vi "CAlex2_rtDisplay.vi"(8 "Cloest Pt":dbl[](array[numeric]), 9 "PrevTraj":dbl[][](array[numeric]), 10 "TargetTraj":dbl[][](array[numeric]), 11 "JointLoc":dbl[][](array[numeric])) -> (3 "new picture":picture)   [LabVIEW 2016, in "CAlex2.lvclass"]
uses:
  CAlex2/CAlex2.lvclass
panel:
  in  "Scale (1) and Offset (0,0)":cluster{"x":i16, "y":i16, "Scale":dbl}={"x"=0, "y"=0, "Scale"=1.0}
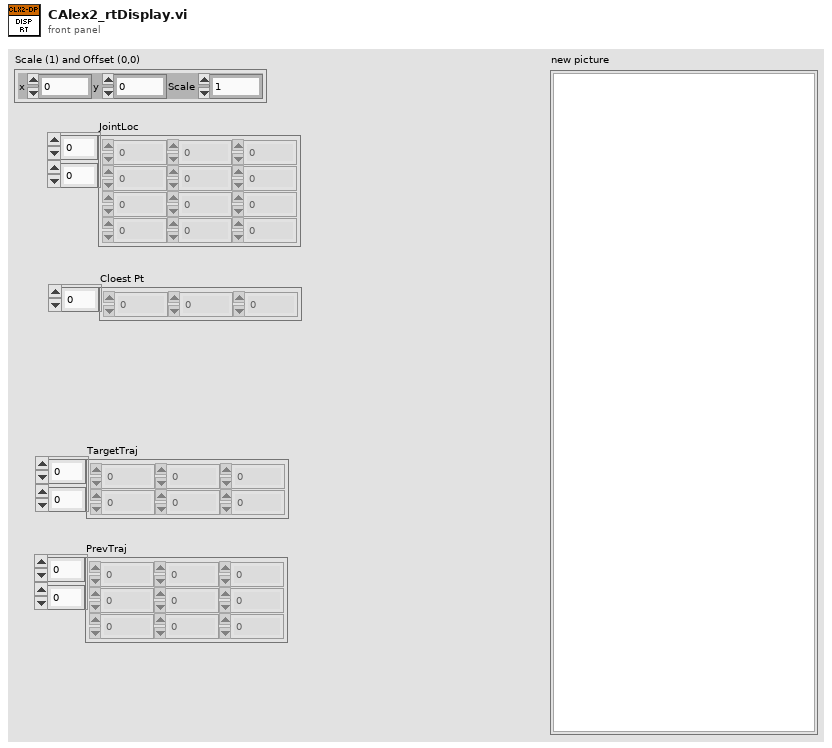
[diagram p1: front panel]
types:
  T1 = cluster{"Width":u16, "Style":enum32{"Solid", "Dash", "Dot", "DashDot", "DashDotDot"}}
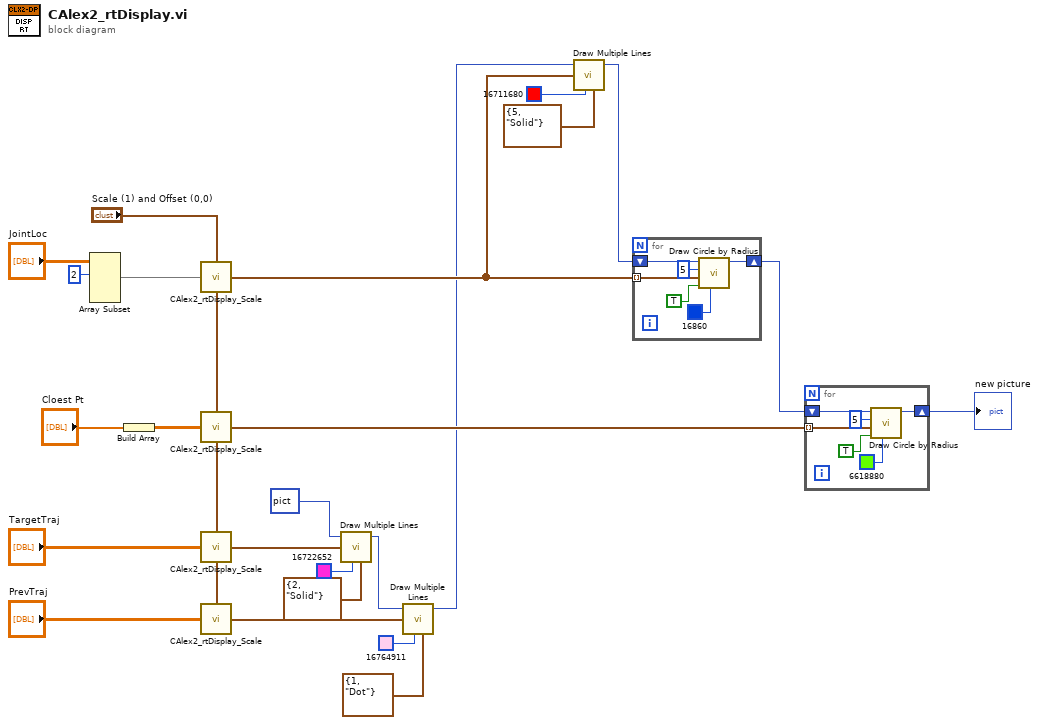
[diagram p0: block diagram]
diagram:
  n1 = Array Subset(array="JointLoc", index (row)=2 ("index")) -> (w9:dbl[][])  [unwired: 3 in]
  n2 = Build Array("Cloest Pt") -> (w6:dbl[][])
  n3 = call "CAlex2_rtDisplay_Scale.vi"("Scale (1) and Offset (0,0)"="Scale (1) and Offset (0,0)", "Input XYZ array"=w9) -> ("Output XY array"=w17:cluster{i16, i16}[])  [unwired: 2 in]
  n4 = call "CAlex2_rtDisplay_Scale.vi"("Scale (1) and Offset (0,0)"="Scale (1) and Offset (0,0)", "Input XYZ array"=w6) -> ("Output XY array"=w5:cluster{i16, i16}[])  [unwired: 2 in]
  n5 = call "CAlex2_rtDisplay_Scale.vi"("Scale (1) and Offset (0,0)"="Scale (1) and Offset (0,0)", "Input XYZ array"="TargetTraj") -> ("Output XY array"=w22:cluster{i16, i16}[])  [unwired: 2 in]
  n6 = call "CAlex2_rtDisplay_Scale.vi"("Scale (1) and Offset (0,0)"="Scale (1) and Offset (0,0)", "Input XYZ array"="PrevTraj") -> ("Output XY array"=w21:cluster{i16, i16}[])  [unwired: 2 in]
  n7 = call <vilib>:"Draw Multiple Lines.vi"("picture"=picture data[5B] ("blank picture"), "line endpoints"=w22, "color(black)"=u32 16722652, "pen"=T1 {"Width"=2, "Style"=enum."Solid"}) -> ("new picture"=w20:picture)  [unwired: 5 in]
  n8 = call <vilib>:"Draw Multiple Lines.vi"("picture"=w20, "line endpoints"=w21, "color(black)"=u32 16764911, "pen"=T1 {"Width"=1, "Style"=enum."Dot"}) -> ("new picture"=w2:picture)  [unwired: 5 in]
  n9 = call <vilib>:"Draw Multiple Lines.vi"("picture"=w2, "line endpoints"=w17, "color(black)"=u32 16711680, "pen"=T1 {"Width"=5, "Style"=enum."Solid"}) -> ("new picture"=w16:picture)  [unwired: 5 in]
  n10 = for {
    tunnel: w17 -> [w30] mode=indexing
    shift-right: [w28] -> w4
    shift-left: w16 -> [w29]
    n11 = call <vilib>:"Draw Circle by Radius.vi"("color(black)"=u32 16860, "fill?(F)"=TRUE, "pixel center"=w30, "radius"=i16 5, "picture"=w29) -> ("new picture"=w28:picture)  [unwired: 6 in]
  }
  n12 = for {
    tunnel: w5 -> [w36] mode=indexing
    shift-right: [w34] -> w1
    shift-left: w4 -> [w35]
    n13 = call <vilib>:"Draw Circle by Radius.vi"("color(black)"=u32 6618880, "fill?(F)"=TRUE, "pixel center"=w36, "radius"=i16 5, "picture"=w35) -> ("new picture"=w34:picture)  [unwired: 6 in]
  }
  "new picture" <- w1
